vi "Read Details.vi"(11 "Protected Actor Handle in":refnum<class "Protected Actor Handle.lvclass">) -> (2 "Actor Details":T1)   [LabVIEW 2020, in "Actor Framework.lvlib" / "Protected Actor Handle.lvclass"]
doc: "Reads identification information about the actor, useful for display in a debugger."
uses:
  Protected Actor Handle.lvclass
  Protected Actor Handle.lvclass/Protected Actor Handle.ctl
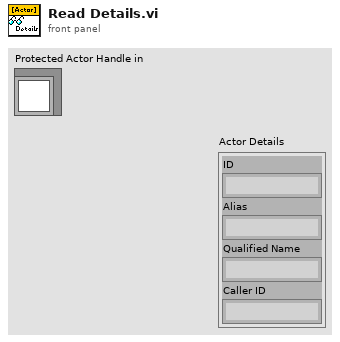
[diagram p1: front panel]
types:
  T1 = cluster{"ID":string, "Alias":string, "Qualified Name":string, "Caller ID":string}
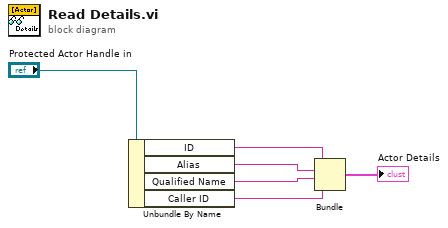
[diagram p0: block diagram]
diagram:
  n1 = Unbundle By Name("Protected Actor Handle in") -> ("ID"=w5:string, "Alias"=w4:string, "Qualified Name"=w2:string, "Caller ID"=w3:string)
  n2 = Bundle("ID"=w5, "Alias"=w4, "Qualified Name"=w2, "Caller ID"=w3) -> (→"Actor Details":T1)  [unwired: 1 in]
